vi "tui_Datalog Tag Subset Editor.vi"() -> ()   [LabVIEW 2012]
doc: "Edits subsets of the collection of tags in a logging database. Tag subsets allow related tags to be grouped. The subsets are ordered. It is possible to reorder the tags in a subset by dragging the items of the \"tags\" list that displays them. Several user interface windows that display information of multiple tags allow these tags to be quickly specified through selection of a subset.\n\nNote that subset definitions are automatically kept in sync with changes to the logging database: when tags that occur in subsets are deleted or renamed, the affected subsets will be updated accordingly. When this occurs while you are editing subsets, the editor will refuse to save any changes made relative to outdated subsets."
uses:
  served/DataLog Database Infos_srv.ctl
  served/DataLog Databases_srv.ctl
  typedefs/t_DataLog Tag Subset Editor States.ctl
  library/typedefs/t_Library Session Methods.ctl
  typedefs/t_DataLog Tag Info List Methods.ctl
  typedefs/t_Datalog Datebase Modes.ctl
  clientsrv/typedefs/t_ClientSrv Access Levels.ctl
panel:
  in  "reload subsets":bool
  in  "new subset":bool
  in  "rename subset":bool
  in  "delete subset":bool
  in  "sort subsets":bool
  in  "subsets":i32(listbox)
  in  "tags":i32(listbox)
  in  "add tag":bool
  in  "add multiple tags":bool
  in  "remove tag":bool
  in  "sort tags":bool
  out "databases":T1
  in  "database":i32(ring)
  in  "save subsets":bool
  in  "exit":bool
  out "database infos":T2
  in  "undo":bool
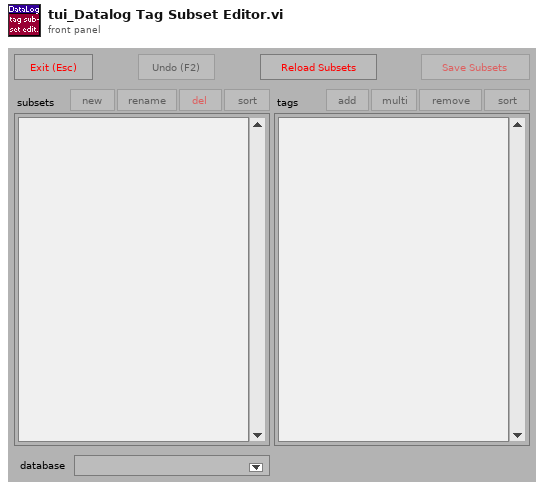
[diagram p1: front panel]
types:
  T1 = typedef "DataLog Databases_srv.ctl" = refnum<vi>
  T2 = typedef "DataLog Database Infos_srv.ctl" = refnum<vi>
  T3 = typedef "t_DataLog Tag Subset Editor States.ctl" = enum16{"empty queue", "set database", "load subsets", "save subsets", "new subset", "rename subset", "delete subset", "sort subsets", "add tag", "add tags", "remove tag", "sort tags", "update lists", "ablement", "resize", "initialize", "init refs", "init databases", "init access", "init persist", "cleanup", "stop"}
  T4 = typedef "t_Library Session Methods.ctl" = enum16{"run", "get arg", "set arg", "delist", "cleanup?", "start session", "stop session", "list empty?"}
  T5 = typedef "t_DataLog Tag Info List Methods.ctl" = enum16{"initialize", "create", "create empty", "rename", "delete", "test tag", "get", "get by name", "get default", "get list", "get path", "get subsets", "set subsets", "set config", "set capacity", "#tags", "go live", "set unlocked", "set mirrored"}
  T6 = typedef "t_Datalog Datebase Modes.ctl" = enum16{"locked", "unlocked", "live", "mirrored"}
  T7 = typedef "t_ClientSrv Access Levels.ctl" = enum16{"observer", "operator", "local"}
  T8 = typedef "t_DataLog Tag Subset.ctl" = cluster{"name":string, "tags":string[]}
  T9 = typedef "eventvkey.ctl" = enum16{"ASCII", "Enter", "Return", "Shift", "Ctrl", "Alt", "Cmd", "Opt", "Caps", "NumLock", "Clear", "Break", "Up", "Down", "Left", "Right", "Insert", "Delete", "Home", "End", "PageUp", "PageDown", "Escape", "Help", "Pause", "ScrollLock", "F1", "F2", "F3", "F4", "F5", "F6", "F7", "F8", "F9", "F10", "F11", "F12", "F13", "F14", "F15", "F16", "F17", "F18", "F19", "F20", "F21", "F22", "F23", "F24", "Play", "VolumeUp", "VolumeDown", "Mute", "Two Byte Char"}
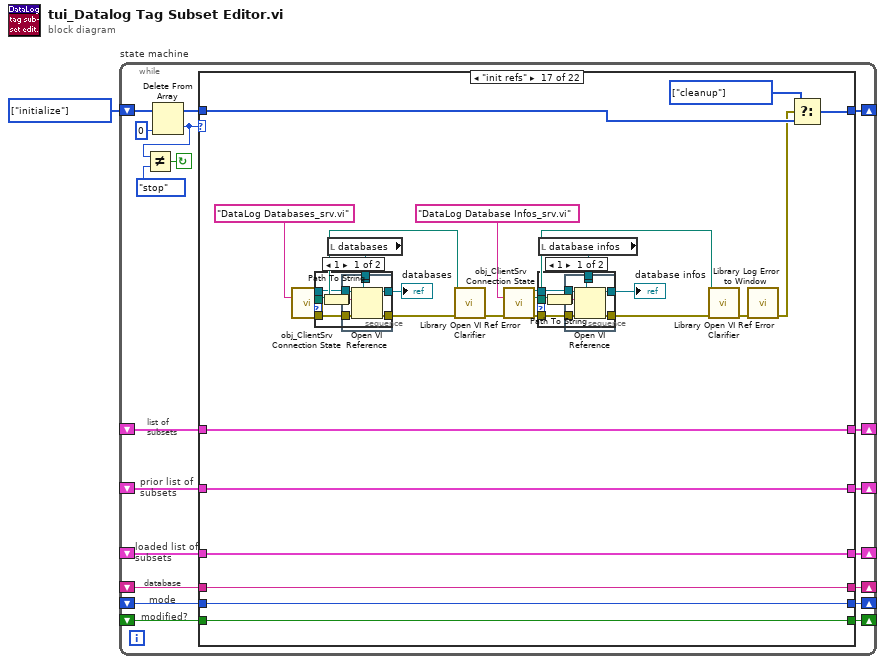
[diagram p0: block diagram]
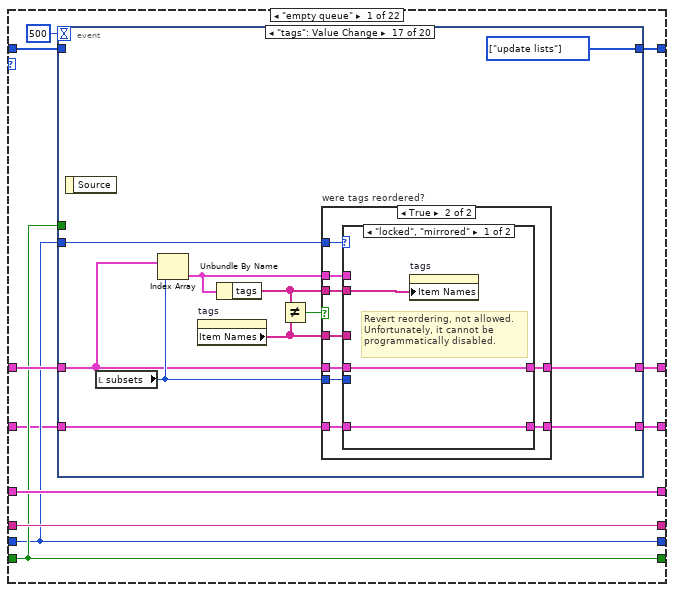
[diagram p2: hidden frame]
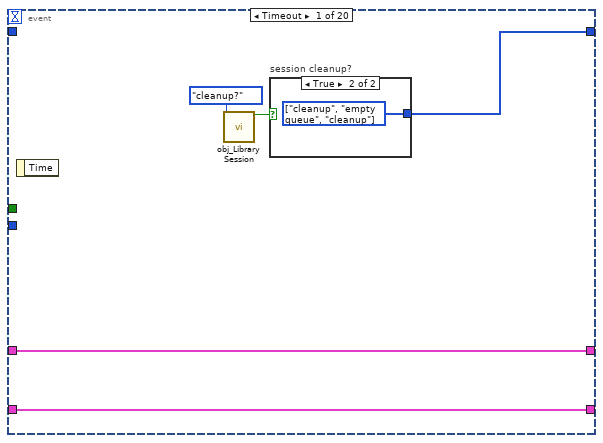
[diagram p3: hidden frame]
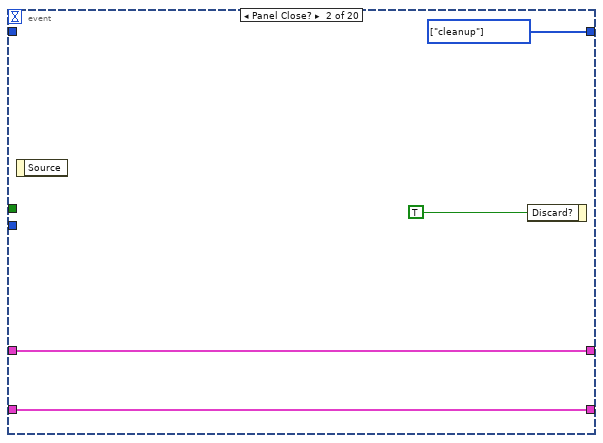
[diagram p5: hidden frame]
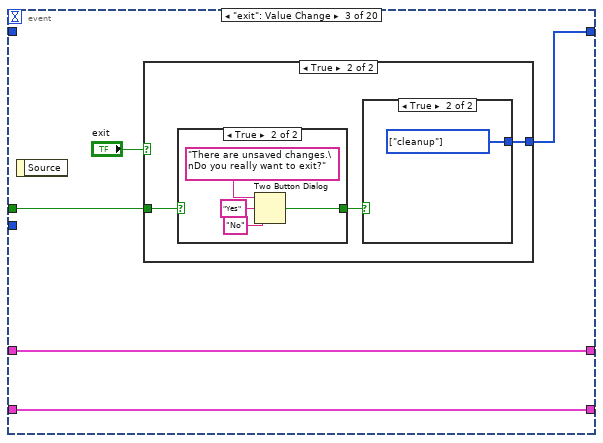
[diagram p6: hidden frame]
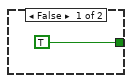
[diagram p8: hidden frame]
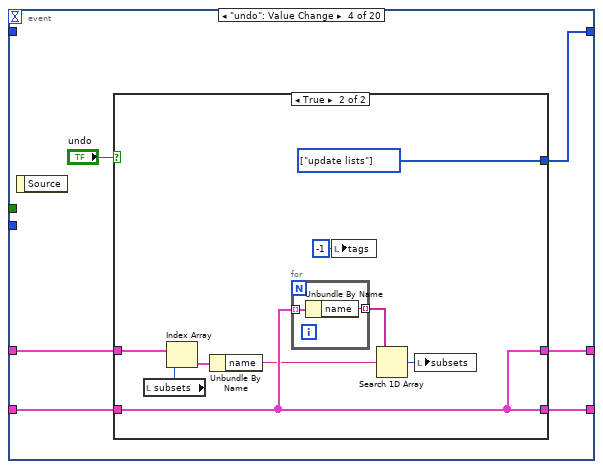
[diagram p10: hidden frame]
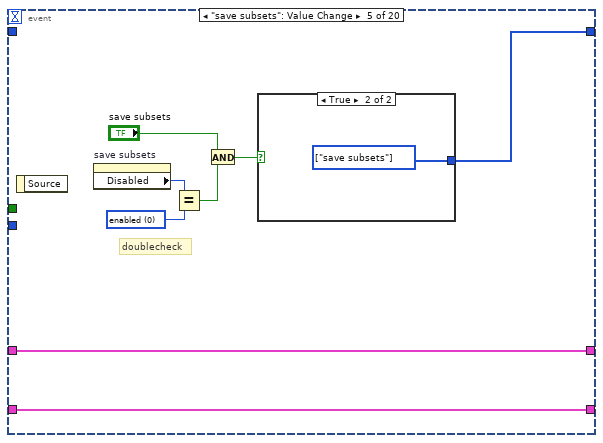
[diagram p12: hidden frame]
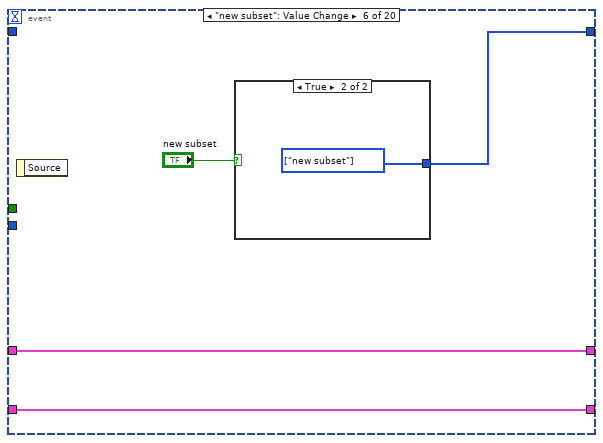
[diagram p14: hidden frame]
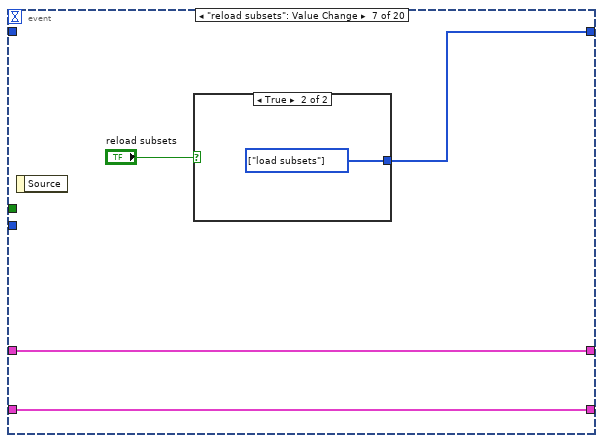
[diagram p16: hidden frame]
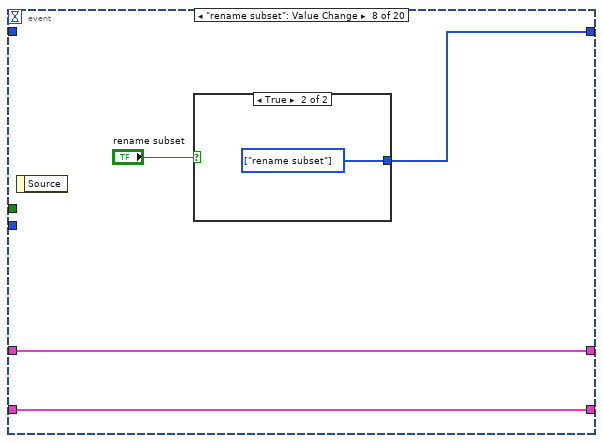
[diagram p18: hidden frame]
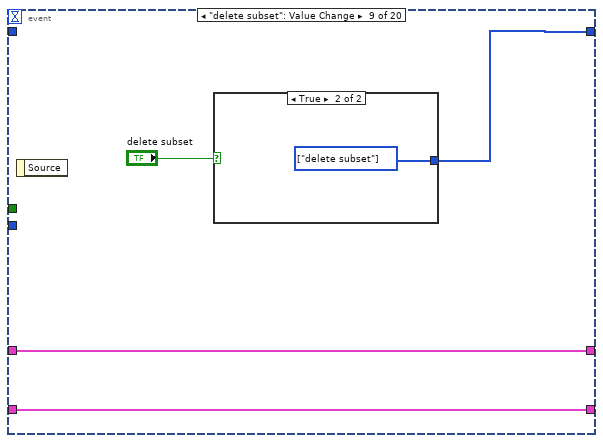
[diagram p20: hidden frame]
diagram:
  w1 = T3[] [enum."initialize"] items=["empty queue", "set database", "load subsets", "save subsets", "new subset", "rename subset", "delete subset", "sort subsets", "add tag", "add tags", "remove tag", "sort tags", "update lists", "ablement", "resize", "initialize", "init refs", "init databases", "init access", "init persist", "cleanup", "stop"] ("Array Constant")
  n1 = while "state machine" {
    shift-left: w1 -> [w17]
    shift-right: [w20] -> _
    shift-right: [w14] -> _
    shift-left: _ -> [w13]
    shift-right: [w10] -> _
    shift-left: _ -> [w11]
    shift-right: [w9] -> _
    shift-left: _ -> [w8]
    shift-right: [w7] -> _
    shift-left: _ -> [w6]
    shift-right: [w5] -> _
    shift-left: _ -> [w4]
    shift-right: [w3] -> _
    shift-left: _ -> [w2]
    stop <- w19 continue-if-true
    # "prior list of\nsubsets"
    # "modified?"
    # "mode"
    # "loaded list of\nsubsets"
    # "database"
    # "list of\nsubsets"
    n2 = Delete From Array(array=w17, index=0) -> (deleted portion=w12:T3, array with subset deleted=w16:T3[])  [unwired: 1 in]
    n3 = Not Equal?(x=w12, y=t_DataLog_Tag_Subset_Editor_States."stop" ("states")) -> (x != y?=w19:bool)
    n4 = case "Case" shown="\"init refs\"" w12 {
      tunnel: [w31 w227 w239 w286 w318 w374 w426 w437 w461 w504 w569 w589 w606 w657 w662 w733 w784 w837 w855 w859 w883 w890] -> w20
      tunnel: w16 -> [w29 w227 w240 w287 w319 w375 w427 w438 w462 w505 w570 w593 w613 w657 w662 _ w783 w827 w854 w865 _ w890]
      tunnel: [w27 w226 w236 w270 w320 w376 w428 w434 w469 w512 w556 w573 w603 w628 w661 w732 w781 w839 w857 w867 w881 w889] -> w14
      tunnel: w13 -> [w28 w226 _ w270 w325 w369 w429 w432 w470 w513 w558 w572 w603 w628 w661 w732 w781 w839 w857 w867 w881 w889]
      tunnel: w11 -> [w26 _ w235 w276 w317 w373 w425 w443 w460 w503 w568 w584 w608 w656 w666 w731 w777 w828 w849 w864 w876 w888]
      tunnel: [w26 w220 w235 w276 w317 w373 w425 w443 w460 w503 w568 w584 w608 w656 w666 w731 w777 w828 w849 w864 w876 w888] -> w10
      tunnel: [w25 w230 w236 w289 w316 w372 w424 w442 w466 w509 w566 w583 w604 w655 w665 w730 w774 w834 w852 w863 w873 w887] -> w9
      tunnel: w8 -> [w25 w230 _ w277 w316 w372 w424 w442 w466 w509 w566 w583 w604 w655 w665 w730 w774 w834 w852 w863 w873 w887]
      tunnel: [w23 w229 w241 w291 w315 w371 w423 w441 w465 w508 w565 w582 w607 w654 w664 w729 w773 w833 w851 w862 w872 w886] -> w7
      tunnel: w6 -> [w23 w229 _ w291 w315 w371 w423 w441 w465 w508 w565 w582 w607 w654 w664 w729 w773 w833 w851 w862 w872 w886]
      tunnel: [w24 w228 FALSE w290 w314 w370 w422 w440 w464 w507 w564 w581 w600 w646 w663 w728 w772 w832 w850 w861 w871 w885] -> w5
      tunnel: w4 -> [w24 w228 w237 w290 w314 w370 w422 w440 w464 w507 w564 w581 w602 w646 w663 w728 w772 w832 w850 w861 w871 w885]
      tunnel: [w21 w225 w236 w273 w313 w363 w420 w435 w459 w502 w560 w575 w599 w630 w660 w727 w771 w831 w846 w860 w868 w884] -> w3
      tunnel: w2 -> [w22 w225 _ w271 w312 w362 w421 w431 w458 w501 w559 w574 w599 w630 w660 w727 w771 w831 w846 w860 w868 w884]
      frame "empty queue" {
        n5 = event shown="[16] \"tags\": Value Change" {
          selector: _ -> [_ _ _ _ _ _ _ _ _ _ _ _ _ _ _ _ _ _ _ _]
          dyn-events: _ -> [_ _ _ _ _ _ _ _ _ _ _ _ _ _ _ _ _ _ _ _]
          timeout: 500 -> [_ _ _ _ _ _ _ _ _ _ _ _ _ _ _ _ _ _ _ _]
          tunnel: [w36 w41 w46 w61 w82 w87 w92 w97 w102 w107 w112 w117 w121 w126 w133 w150 w181 _ _ w217] -> w31
          tunnel: w29 -> [_ _ _ _ _ _ _ _ _ _ _ _ _ _ _ _ _ _ _ _]
          tunnel: w28 -> [w33 w39 w45 w56 w81 w86 w91 w96 w101 w106 w111 w116 w122 w127 w134 w147 w182 w207 w213 w219]
          tunnel: [w33 w39 w45 w59 w81 w86 w91 w96 w101 w106 w111 w116 w122 w127 w134 w145 w184 w207 w213 w219] -> w27
          tunnel: w24 -> [_ _ w43 _ _ _ _ _ _ _ _ _ _ _ w132 _ _ _ _ _]
          tunnel: w23 -> [_ _ _ _ _ _ _ _ _ _ _ _ _ _ _ w144 w176 _ _ _]
          tunnel: w22 -> [w32 w38 w42 w58 w80 w84 w89 w94 w99 w104 w109 w114 w119 w124 w129 w141 w174 w206 w212 w218]
          tunnel: [w32 w38 w42 w57 w80 w84 w89 w94 w99 w104 w109 w114 w119 w124 w129 w142 w175 w206 w212 w218] -> w21
          event Timeout {
            n6 = event-data() -> ()  [unwired: 1 in, 1 out]
            n7 = call "obj_Library Session.vi"("method"=t_Library_Session_Methods."cleanup?") -> ("cleanup/empty?"=w35:bool)  [unwired: 11 in, 3 out]
            n8 = case "session cleanup?" shown="True" w35 {
              tunnel: [_ w37] -> w36
              frame False {
              }
              frame True {
                w37 = T3[] [enum."cleanup", enum."empty queue", enum."cleanup"] items=["empty queue", "set database", "load subsets", "save subsets", "new subset", "rename subset", "delete subset", "sort subsets", "add tag", "add tags", "remove tag", "sort tags", "update lists", "ablement", "resize", "initialize", "init refs", "init databases", "init access", "init persist", "cleanup", "stop"] ("Array Constant")
              }
            }
          }
          event Panel Close? {
            w41 = T3[] [enum."cleanup"] items=["empty queue", "set database", "load subsets", "save subsets", "new subset", "rename subset", "delete subset", "sort subsets", "add tag", "add tags", "remove tag", "sort tags", "update lists", "ablement", "resize", "initialize", "init refs", "init databases", "init access", "init persist", "cleanup", "stop"] ("Array Constant")
            n9 = event-data() -> ()  [unwired: 1 in, 1 out]
            n10 = event-data("Discard?"=TRUE) -> ()  [unwired: 1 in, 1 out]
          }
          event "exit": Value Change {
            n11 = event-data() -> ()  [unwired: 1 in, 1 out]
            n12 = case shown="True" "exit" {
              tunnel: [_ w49] -> w46
              tunnel: w43 -> [_ w48]
              frame False {
              }
              frame True {
                n13 = case shown="True" w48 {
                  tunnel: [TRUE w53] -> w47
                  frame False {
                  }
                  frame True {
                    n14 = Two Button Dialog(message="There are unsaved changes.\nDo you really want to exit?", 1:"No" ("F button name (\"Cancel\")"), 2:"Yes" ("T button name (\"OK\")")) -> (T button?=w53:bool)
                  }
                }
                n15 = case shown="True" w47 {
                  tunnel: [_ w55] -> w49
                  frame False {
                  }
                  frame True {
                    w55 = T3[] [enum."cleanup"] items=["empty queue", "set database", "load subsets", "save subsets", "new subset", "rename subset", "delete subset", "sort subsets", "add tag", "add tags", "remove tag", "sort tags", "update lists", "ablement", "resize", "initialize", "init refs", "init databases", "init access", "init persist", "cleanup", "stop"] ("Array Constant")
                  }
                }
              }
            }
          }
          event "undo": Value Change {
            n16 = event-data() -> ()  [unwired: 1 in, 1 out]
            n17 = case shown="True" "undo" {
              tunnel: [_ w72] -> w61
              tunnel: [w63 w68] -> w59
              tunnel: w58 -> [w62 w68]
              tunnel: [w62 w68] -> w57
              tunnel: w56 -> [w63 w71]
              frame False {
              }
              frame True {
                w72 = T3[] [enum."update lists"] items=["empty queue", "set database", "load subsets", "save subsets", "new subset", "rename subset", "delete subset", "sort subsets", "add tag", "add tags", "remove tag", "sort tags", "update lists", "ablement", "resize", "initialize", "init refs", "init databases", "init access", "init persist", "cleanup", "stop"] ("Array Constant")
                n18 = local read "subsets"() -> (w70:i32)
                n19 = Index Array(array=w71, index=w70) -> (element=w69:T8)
                n20 = Unbundle By Name(w69) -> ("name"=w66:string)
                n21 = for {
                  tunnel: w68 -> [w74] mode=indexing
                  tunnel: [w73] -> w67 mode=indexing
                  n22 = Unbundle By Name(w74) -> ("name"=w73:string)
                }
                n23 = local write "tags"(-1 ("tags")) -> ()
                n24 = Search 1D Array(1D array=w67, element=w66) -> (index of element=w65:i32)  [unwired: 1 in]
                n25 = local write "subsets"(w65) -> ()
              }
            }
          }
          event "save subsets": Value Change {
            w79 = u8 0 items=["enabled", "disabled", "grayed"] ("disabled state")
            # "doublecheck"
            n26 = event-data() -> ()  [unwired: 1 in, 1 out]
            n27 = property on="save subsets" class="Bool"() -> ("Disabled"=w78:u8)  [unwired: 2 in, 2 out]
            n28 = Equal?(x=w78, y=w79) -> (x = y?=w76:bool)
            n29 = And(x="save subsets", y=w76) -> (x .and. y?=w75:bool)
            n30 = case shown="True" w75 {
              tunnel: [_ w83] -> w82
              frame False {
              }
              frame True {
                w83 = T3[] [enum."save subsets"] items=["empty queue", "set database", "load subsets", "save subsets", "new subset", "rename subset", "delete subset", "sort subsets", "add tag", "add tags", "remove tag", "sort tags", "update lists", "ablement", "resize", "initialize", "init refs", "init databases", "init access", "init persist", "cleanup", "stop"] ("Array Constant")
              }
            }
          }
          event "new subset": Value Change {
            n31 = event-data() -> ()  [unwired: 1 in, 1 out]
            n32 = case shown="True" "new subset" {
              tunnel: [_ w88] -> w87
              frame False {
              }
              frame True {
                w88 = T3[] [enum."new subset"] items=["empty queue", "set database", "load subsets", "save subsets", "new subset", "rename subset", "delete subset", "sort subsets", "add tag", "add tags", "remove tag", "sort tags", "update lists", "ablement", "resize", "initialize", "init refs", "init databases", "init access", "init persist", "cleanup", "stop"] ("Array Constant")
              }
            }
          }
          event "reload subsets": Value Change {
            n33 = event-data() -> ()  [unwired: 1 in, 1 out]
            n34 = case shown="True" "reload subsets" {
              tunnel: [_ w93] -> w92
              frame False {
              }
              frame True {
                w93 = T3[] [enum."load subsets"] items=["empty queue", "set database", "load subsets", "save subsets", "new subset", "rename subset", "delete subset", "sort subsets", "add tag", "add tags", "remove tag", "sort tags", "update lists", "ablement", "resize", "initialize", "init refs", "init databases", "init access", "init persist", "cleanup", "stop"] ("Array Constant")
              }
            }
          }
          event "rename subset": Value Change {
            n35 = event-data() -> ()  [unwired: 1 in, 1 out]
            n36 = case shown="True" "rename subset" {
              tunnel: [_ w98] -> w97
              frame False {
              }
              frame True {
                w98 = T3[] [enum."rename subset"] items=["empty queue", "set database", "load subsets", "save subsets", "new subset", "rename subset", "delete subset", "sort subsets", "add tag", "add tags", "remove tag", "sort tags", "update lists", "ablement", "resize", "initialize", "init refs", "init databases", "init access", "init persist", "cleanup", "stop"] ("Array Constant")
              }
            }
          }
          event "delete subset": Value Change {
            n37 = event-data() -> ()  [unwired: 1 in, 1 out]
            n38 = case shown="True" "delete subset" {
              tunnel: [_ w103] -> w102
              frame False {
              }
              frame True {
                w103 = T3[] [enum."delete subset"] items=["empty queue", "set database", "load subsets", "save subsets", "new subset", "rename subset", "delete subset", "sort subsets", "add tag", "add tags", "remove tag", "sort tags", "update lists", "ablement", "resize", "initialize", "init refs", "init databases", "init access", "init persist", "cleanup", "stop"] ("Array Constant")
              }
            }
          }
          event "remove tag": Value Change {
            n39 = event-data() -> ()  [unwired: 1 in, 1 out]
            n40 = case shown="True" "remove tag" {
              tunnel: [_ w108] -> w107
              frame False {
              }
              frame True {
                w108 = T3[] [enum."remove tag"] items=["empty queue", "set database", "load subsets", "save subsets", "new subset", "rename subset", "delete subset", "sort subsets", "add tag", "add tags", "remove tag", "sort tags", "update lists", "ablement", "resize", "initialize", "init refs", "init databases", "init access", "init persist", "cleanup", "stop"] ("Array Constant")
              }
            }
          }
          event "add tag": Value Change {
            n41 = event-data() -> ()  [unwired: 1 in, 1 out]
            n42 = case shown="True" "add tag" {
              tunnel: [_ w113] -> w112
              frame False {
              }
              frame True {
                w113 = T3[] [enum."add tag"] items=["empty queue", "set database", "load subsets", "save subsets", "new subset", "rename subset", "delete subset", "sort subsets", "add tag", "add tags", "remove tag", "sort tags", "update lists", "ablement", "resize", "initialize", "init refs", "init databases", "init access", "init persist", "cleanup", "stop"] ("Array Constant")
              }
            }
          }
          event "add multiple tags": Value Change {
            n43 = event-data() -> ()  [unwired: 1 in, 1 out]
            n44 = case shown="True" "add multiple tags" {
              tunnel: [_ w118] -> w117
              frame False {
              }
              frame True {
                w118 = T3[] [enum."add tags"] items=["empty queue", "set database", "load subsets", "save subsets", "new subset", "rename subset", "delete subset", "sort subsets", "add tag", "add tags", "remove tag", "sort tags", "update lists", "ablement", "resize", "initialize", "init refs", "init databases", "init access", "init persist", "cleanup", "stop"] ("Array Constant")
              }
            }
          }
          event "sort tags": Value Change {
            n45 = event-data() -> ()  [unwired: 1 in, 1 out]
            n46 = case shown="True" "sort tags" {
              tunnel: [_ w123] -> w121
              frame False {
              }
              frame True {
                w123 = T3[] [enum."sort tags"] items=["empty queue", "set database", "load subsets", "save subsets", "new subset", "rename subset", "delete subset", "sort subsets", "add tag", "add tags", "remove tag", "sort tags", "update lists", "ablement", "resize", "initialize", "init refs", "init databases", "init access", "init persist", "cleanup", "stop"] ("Array Constant")
              }
            }
          }
          event "sort subsets": Value Change {
            n47 = event-data() -> ()  [unwired: 1 in, 1 out]
            n48 = case shown="True" "sort subsets" {
              tunnel: [_ w128] -> w126
              frame False {
              }
              frame True {
                w128 = T3[] [enum."sort subsets"] items=["empty queue", "set database", "load subsets", "save subsets", "new subset", "rename subset", "delete subset", "sort subsets", "add tag", "add tags", "remove tag", "sort tags", "update lists", "ablement", "resize", "initialize", "init refs", "init databases", "init access", "init persist", "cleanup", "stop"] ("Array Constant")
              }
            }
          }
          event "database": Value Change {
            n49 = event-data() -> ("OldVal"=w130:i32)  [unwired: 1 in]
            n50 = case shown="False" w132 {
              tunnel: [TRUE w138] -> w131
              frame False {
              }
              frame True {
                n51 = Two Button Dialog(message="You have selected a new database\nbut the prior database has unsaved\nsubset changes. If you proceed,\nthese changes will be discarded.", 2:"Proceed" ("T button name (\"OK\")")) -> (T button?=w138:bool)  [unwired: 1 in]
              }
            }
            n52 = case shown="True" w131 {
              tunnel: [_ w140] -> w133
              tunnel: w130 -> [w139 _]
              frame False {
                n53 = local write "database"(w139) -> ()
              }
              frame True {
                w140 = T3[] [enum."set database", enum."load subsets"] items=["empty queue", "set database", "load subsets", "save subsets", "new subset", "rename subset", "delete subset", "sort subsets", "add tag", "add tags", "remove tag", "sort tags", "update lists", "ablement", "resize", "initialize", "init refs", "init databases", "init access", "init persist", "cleanup", "stop"] ("Array Constant")
              }
            }
          }
          event "subsets": Value Change {
            w150 = T3[] [enum."update lists"] items=["empty queue", "set database", "load subsets", "save subsets", "new subset", "rename subset", "delete subset", "sort subsets", "add tag", "add tags", "remove tag", "sort tags", "update lists", "ablement", "resize", "initialize", "init refs", "init databases", "init access", "init persist", "cleanup", "stop"] ("Array Constant")
            n54 = event-data() -> ()  [unwired: 1 in, 1 out]
            n55 = for {
              tunnel: w147 -> [w173] mode=indexing
              tunnel: [w172] -> w146 mode=indexing
              n56 = Unbundle By Name(w173) -> ("name"=w172:string)
            }
            n57 = property on="subsets" class="LstBox (strict)"() -> ("Item Names"=w148:string[])  [unwired: 2 in, 2 out]
            n58 = Not Equal?(x=w148, y=w146) -> (x != y?=w149:bool)
            n59 = case "were subsets reordered?" shown="True" w149 {
              tunnel: w148 -> [_ w159]
              tunnel: w147 -> [w152 w157]
              tunnel: w146 -> [_ w158]
              tunnel: [w152 w156] -> w145
              tunnel: w144 -> [_ w155]
              tunnel: [w151 w154] -> w142
              tunnel: w141 -> [w151 w153]
              frame False {
              }
              frame True {
                n60 = case shown="\"locked\", \"mirrored\"" w155 {
                  tunnel: w159 -> [_ w166]
                  tunnel: w158 -> [w161 w165]
                  tunnel: w157 -> [w162 w163]
                  tunnel: [w162 w164] -> w156
                  tunnel: [w160 w163] -> w154
                  tunnel: w153 -> [w160 _]
                  frame "locked", "mirrored" {
                    # "Revert reordering, not allowed.\nUnfortunately, it cannot be\nprogrammatically disabled."
                    n61 = property on="subsets" class="LstBox (strict)"("Item Names"=w161) -> ()  [unwired: 2 in, 2 out]
                  }
                  frame "unlocked", "live" {
                    n62 = for {
                      tunnel: w166 -> [w170] mode=indexing
                      tunnel: w165 -> [w171]
                      tunnel: w163 -> [w168]
                      tunnel: [w167] -> w164 mode=indexing
                      n63 = Search 1D Array(1D array=w171, element=w170) -> (index of element=w169:i32)  [unwired: 1 in]
                      n64 = Index Array(array=w168, index=w169) -> (element=w167:T8)
                    }
                  }
                }
              }
            }
            n65 = local write "tags"(-1 ("list of tag subsets")) -> ()
          }
          event "tags": Value Change {
            w181 = T3[] [enum."update lists"] items=["empty queue", "set database", "load subsets", "save subsets", "new subset", "rename subset", "delete subset", "sort subsets", "add tag", "add tags", "remove tag", "sort tags", "update lists", "ablement", "resize", "initialize", "init refs", "init databases", "init access", "init persist", "cleanup", "stop"] ("Array Constant")
            n66 = event-data() -> ()  [unwired: 1 in, 1 out]
            n67 = local read "subsets"() -> (w183:i32)
            n68 = Index Array(array=w182, index=w183) -> (element=w179:T8)
            n69 = property on="tags" class="LstBox (strict)"() -> ("Item Names"=w178:string[])  [unwired: 2 in, 2 out]
            n70 = Unbundle By Name(w179) -> ("tags"=w177:string[])
            n71 = Not Equal?(x=w177, y=w178) -> (x != y?=w180:bool)
            n72 = case "were tags reordered?" shown="True" w180 {
              tunnel: [w186 w195] -> w184
              tunnel: w183 -> [_ w194]
              tunnel: w182 -> [w186 w193]
              tunnel: w179 -> [_ w192]
              tunnel: w178 -> [_ w191]
              tunnel: w177 -> [_ w190]
              tunnel: w176 -> [_ w189]
              tunnel: [w185 w188] -> w175
              tunnel: w174 -> [w185 w187]
              frame False {
              }
              frame True {
                n73 = case shown="\"locked\", \"mirrored\"" w189 {
                  tunnel: [w198 w204] -> w195
                  tunnel: w194 -> [_ w203]
                  tunnel: w193 -> [w198 w199]
                  tunnel: w192 -> [_ w201]
                  tunnel: w191 -> [_ w200]
                  tunnel: w190 -> [w197 _]
                  tunnel: [w196 w199] -> w188
                  tunnel: w187 -> [w196 _]
                  frame "locked", "mirrored" {
                    # "Revert reordering, not allowed.\nUnfortunately, it cannot be\nprogrammatically disabled."
                    n74 = property on="tags" class="LstBox (strict)"("Item Names"=w197) -> ()  [unwired: 2 in, 2 out]
                  }
                  frame "unlocked", "live" {
                    n75 = Bundle By Name(cluster=w201, "tags"=w200) -> (w202:T8)
                    n76 = Replace Array Subset(array=w199, new element=w202, index=w203) -> (w204:T8[])
                  }
                }
              }
            }
          }
          event Key Down? {
            n77 = event-data() -> ("VKey"=w205:T9)  [unwired: 1 in]
            n78 = call <vilib>:"compatReturnToEnter.vi"("VKey"=w205) -> ("VKey"=w209:T9)
            n79 = case shown="\"F1\"" w209 {
              tunnel: [_ TRUE ("Discard?")] -> w208
              frame Default {
              }
              frame "F1" {
                n80 = call "Library Show Help.vi"() -> ()  [unwired: 1 in]
              }
            }
            n81 = event-data("Discard?"=w208) -> ()  [unwired: 1 in, 1 out]
          }
          event event type 5.0.x8000000b {
            n82 = event-data() -> ("VKey"=w211:T9)  [unwired: 1 in]
            n83 = call <vilib>:"compatReturnToEnter.vi"("VKey"=w211) -> ("VKey"=w215:T9)
            n84 = case shown="\"F1\"" w215 {
              tunnel: [_ TRUE ("Discard?")] -> w214
              frame Default {
              }
              frame "F1" {
              }
            }
            n85 = event-data("Discard?"=w214) -> ()  [unwired: 1 in, 1 out]
          }
          event Panel Resize {
            w217 = T3[] [enum."resize"] items=["empty queue", "set database", "load subsets", "save subsets", "new subset", "rename subset", "delete subset", "sort subsets", "add tag", "add tags", "remove tag", "sort tags", "update lists", "ablement", "resize", "initialize", "init refs", "init databases", "init access", "init persist", "cleanup", "stop"] ("Array Constant")
            n86 = event-data() -> ()  [unwired: 1 in, 1 out]
          }
        }
      }
      frame "set database" {
        n87 = property on="database" class="Ring (strict)"() -> ("Strings []"=w221:string[])  [unwired: 2 in, 2 out]
        n88 = Index Array(array=w221, index="database") -> (element=w222:string)
        n89 = Empty String/Path?(string/path=w222) -> (empty?=w223:bool)
        n90 = case shown="True" w223 {
          tunnel: w221 -> [_ w234]
          tunnel: w222 -> [w231 _]
          tunnel: [w231 w233] -> w220
          frame False {
          }
          frame True {
            w232 = 0 ("index")
            n91 = Index Array(array=w234, index=w232) -> (element=w233:string)
            n92 = local write "database"(w232) -> ()
          }
        }
      }
      frame "load subsets" {
        n93 = call "obj_ClientSrv Client Access State.vi"() -> ("certificate"=w246:string, "error out"=w250:errorcluster)  [unwired: 14 in]
        n94 = local read "database infos"() -> (w247:T2)
        n95 = call-by-ref "?"(reference=w247, error in=w250, "method"=t_DataLog_Tag_Info_List_Methods."get subsets", "certificate in"=w246, "database (current)"=w235) -> (error out=w249:errorcluster, "mode"=w244:T6, "subsets out"=w242:T8[], 15:"error out"=w248:errorcluster)  [unwired: 7 in, 4 out]
        n96 = call "Library Remote Call Error Merger.vi"("call by reference node error"=w249, "called VI error (no error)"=w248) -> ("error out"=w243:errorcluster)  [unwired: 13 in]
        n97 = case shown="No Error" w243 {
          selector: w243 -> [_ w268]
          tunnel: w244 -> [w259 _]
          tunnel: w242 -> [w258 _]
          tunnel: [w258 _] -> w236
          tunnel: [w257 t_Datalog_Datebase_Modes."locked" ("mode")] -> w241
          tunnel: w240 -> [w256 _]
          tunnel: [w255 w267] -> w239
          tunnel: w237 -> [w251 _]
          frame No Error {
            n98 = case shown="\"locked\", \"mirrored\"" w259 {
              selector: w259 -> [w262 w266]
              tunnel: [w262 w266] -> w257
              tunnel: [-1 ("list of tag subsets") 0 ("list of tag subsets")] -> w252
              frame "locked", "mirrored" {
                n99 = Format Into String(format string="Database is %s. Can view\nbut not edit its tag subsets.", w262) -> (resulting string=w263:string)  [unwired: 2 in, 1 out]
                n100 = One Button Dialog(message=w263) -> ()  [unwired: 1 in, 1 out]
              }
              frame "unlocked", "live" {
              }
            }
            n101 = case shown="True" w251 {
              frame False {
              }
              frame True {
                n102 = property class="VI"("Front Panel Window:Title"="Tag Subset Editor") -> ()  [unwired: 2 in, 2 out]
              }
            }
            n103 = local write "tags"(-1 ("list of tag subsets")) -> ()
            n104 = local write "subsets"(w252) -> ()
            n105 = Build Array (concatenate)(t_DataLog_Tag_Subset_Editor_States."update lists" ("states"), w256) -> (w255:T3[])
          }
          frame Error {
            w267 = T3[] [enum."cleanup"] items=["empty queue", "set database", "load subsets", "save subsets", "new subset", "rename subset", "delete subset", "sort subsets", "add tag", "add tags", "remove tag", "sort tags", "update lists", "ablement", "resize", "initialize", "init refs", "init databases", "init access", "init persist", "cleanup", "stop"] ("Array Constant")
            n106 = call "Library Log Error to Window.vi"("error in (no error)"=w268) -> ()  [unwired: 13 in, 2 out]
          }
        }
      }
      frame "save subsets" {
        n107 = local read "database infos"() -> (w282:T2)
        n108 = call "obj_ClientSrv Client Access State.vi"() -> ("certificate"=w284:string, "error out"=w283:errorcluster)  [unwired: 14 in]
        n109 = call-by-ref "?"(reference=w282, error in=w283, "method"=t_DataLog_Tag_Info_List_Methods."get subsets", "certificate in"=w284, "database (current)"=w276) -> (reference out=w281:T2, error out=w280:errorcluster, "subsets out"=w278:T8[], 15:"error out"=w279:errorcluster)  [unwired: 7 in, 4 out]
        n110 = Equal?(x=w278, y=w277) -> (x = y?=w274:bool)
        n111 = call "Library Remote Call Error Merger.vi"("call by reference node error"=w280, "called VI error (no error)"=w279) -> ("error out"=w275:errorcluster)  [unwired: 13 in]
        n112 = case shown="No Error" w275 {
          selector: w275 -> [_ w311]
          tunnel: w270 -> [w296 _]
          tunnel: [w295 w310] -> w272
          tunnel: w281 -> [w294 _]
          tunnel: w276 -> [w293 _]
          tunnel: w274 -> [w292 _]
          frame No Error {
            n113 = case "subsets remained unchanged while editing?" shown="True" w292 {
              tunnel: w293 -> [_ w309]
              tunnel: w296 -> [_ w301]
              tunnel: [TRUE w300] -> w295
              tunnel: w294 -> [_ w299]
              frame False {
                n114 = One Button Dialog(message="Cannot save changes. While editing, the\nsubsets of the database were modified.\nThis can happen when tags are renamed\nor deleted while editing, or another user\nhas edited subsets in the mean time.\n\nFirst reload the subsets to make changes\nagainst to the current definitions.") -> ()  [unwired: 1 in, 1 out]
              }
              frame True {
                n115 = call "obj_ClientSrv Client Access State.vi"("access level (observer)"=t_ClientSrv_Access_Levels."operator") -> ("certificate"=w303:string, "error out"=w308:errorcluster)  [unwired: 13 in]
                n116 = call-by-ref "?"(reference=w299, error in=w308, "method"=t_DataLog_Tag_Info_List_Methods."set subsets", "subsets in"=w301, "certificate in"=w303, "database (current)"=w309) -> (error out=w307:errorcluster, 15:"error out"=w304:errorcluster)  [unwired: 6 in, 6 out]
                n117 = call "Library Remote Call Error Merger.vi"("call by reference node error"=w307, "called VI error (no error)"=w304) -> ("error out"=w306:errorcluster)  [unwired: 13 in]
                n118 = call "Library Log Error to Window.vi"("error in (no error)"=w306) -> ("error?"=w300:bool)  [unwired: 13 in, 1 out]
              }
            }
          }
          frame Error {
            n119 = call "Library Log Error to Window.vi"("error in (no error)"=w311) -> ("error?"=w310:bool)  [unwired: 13 in, 1 out]
          }
        }
        n120 = Build Array (concatenate)(t_DataLog_Tag_Subset_Editor_States."update lists" ("states"), w287) -> (w286:T3[])
        n121 = Select(t=w271, s=w272, f=w270) -> (s? t:f=w273:T8[])
        n122 = Select(t=w277, s=w272, f=w270) -> (s? t:f=w289:T8[])
      }
      frame "new subset" {
        n123 = call "ui_Library Query String.vi"("prompt"="Name the new tag subset") -> ("OKed?"=w324:bool, "string out"=w321:string)  [unwired: 13 in]
        n124 = Empty String/Path?(string/path=w321) -> (empty?=w323:bool)
        n125 = Compound Arithmetic op=AND(w324, invert w323) -> (w322:bool)
        n126 = case shown="True" w322 {
          tunnel: w325 -> [w328 w335]
          tunnel: w321 -> [_ w333]
          tunnel: [w328 w338] -> w320
          tunnel: w319 -> [w329 w337]
          tunnel: [w329 w336] -> w318
          tunnel: [w327 w331] -> w313
          tunnel: w312 -> [w327 w330]
          frame False {
          }
          frame True {
            n127 = for {
              tunnel: w335 -> [w344] mode=indexing
              shift-right: [w339] -> w332
              shift-left: FALSE -> [w343]
              tunnel: w333 -> [w341]
              n128 = Unbundle By Name(w344) -> ("name"=w342:string)
              n129 = Equal?(x=w341, y=w342) -> (x = y?=w340:bool)
              n130 = Or(x=w343, y=w340) -> (x .or. y?=w339:bool)
            }
            n131 = case "exists already?" shown="False" w332 {
              tunnel: w335 -> [w345 w361]
              tunnel: [w355 w361] -> w338
              tunnel: w333 -> [w352 w359]
              tunnel: w337 -> [w347 w360]
              tunnel: [w346 w360] -> w336
              tunnel: [w345 w356] -> w331
              tunnel: w330 -> [_ w356]
              frame False {
                n132 = Index Array(array=w345, index=0) -> (element=w353:T8)
                n133 = Bundle By Name(cluster=w353, "name"=w352, "tags"=string[] []) -> (w350:T8)
                n134 = Array Size(array=w345) -> (size(s)=w349:i32)
                n135 = Build Array (concatenate)(w345, w350) -> (w355:T8[])
                n136 = Build Array (concatenate)(t_DataLog_Tag_Subset_Editor_States."update lists" ("states"), w347) -> (w346:T3[])
                n137 = local write "subsets"(w349) -> ()
              }
              frame True {
                n138 = Format Into String(format string="Subset \"%s\" already exists.", w359) -> (resulting string=w357:string)  [unwired: 2 in, 1 out]
                n139 = One Button Dialog(message=w357) -> ()  [unwired: 1 in, 1 out]
              }
            }
          }
        }
      }
      frame "rename subset" {
        n140 = local read "subsets"() -> (w368:i32)
        n141 = Index Array(array=w369, index=w368) -> (element=w367:T8)
        n142 = Unbundle By Name(w367) -> ("name"=w365:string)
        n143 = call "ui_Library Query String.vi"("prompt"="Specify a new subset name", "string in (\"\")"=w365) -> ("OKed?"=w379:bool, "string out"=w366:string)  [unwired: 12 in]
        n144 = Equal?(x=w366, y=w365) -> (x = y?=w364:bool)
        n145 = Empty String/Path?(string/path=w366) -> (empty?=w378:bool)
        n146 = Compound Arithmetic op=AND(w379, invert w378, invert w364) -> (w377:bool)
        n147 = case "new name OKed?" shown="True" w377 {
          tunnel: w369 -> [w382 w390]
          tunnel: w366 -> [_ w388]
          tunnel: [w382 w393] -> w376
          tunnel: w375 -> [w383 w392]
          tunnel: [w383 w391] -> w374
          tunnel: w368 -> [_ w386]
          tunnel: [w381 w385] -> w363
          tunnel: w362 -> [w381 w384]
          frame False {
          }
          frame True {
            n148 = for {
              tunnel: w390 -> [w399] mode=indexing
              shift-right: [w394] -> w387
              shift-left: FALSE -> [w398]
              tunnel: w388 -> [w396]
              n149 = Unbundle By Name(w399) -> ("name"=w397:string)
              n150 = Equal?(x=w396, y=w397) -> (x = y?=w395:bool)
              n151 = Or(x=w398, y=w395) -> (x .or. y?=w394:bool)
            }
            n152 = case "exists already?" shown="False" w387 {
              tunnel: w390 -> [w400 w414]
              tunnel: [w403 w414] -> w393
              tunnel: w388 -> [w407 w412]
              tunnel: w392 -> [w405 w413]
              tunnel: [w404 w413] -> w391
              tunnel: w386 -> [w401 _]
              tunnel: [w400 w409] -> w385
              tunnel: w384 -> [_ w409]
              frame False {
                n153 = Index Array(array=w400, index=w401) -> (element=w408:T8)
                n154 = Bundle By Name(cluster=w408, "name"=w407) -> (w402:T8)
                n155 = Build Array (concatenate)(t_DataLog_Tag_Subset_Editor_States."update lists" ("states"), w405) -> (w404:T3[])
                n156 = Replace Array Subset(array=w400, new element=w402, index=w401) -> (w403:T8[])
              }
              frame True {
                n157 = Format Into String(format string="Subset \"%s\" already exists.", w412) -> (resulting string=w410:string)  [unwired: 2 in, 1 out]
                n158 = One Button Dialog(message=w410) -> ()  [unwired: 1 in, 1 out]
              }
            }
          }
        }
      }
      frame "delete subset" {
        n159 = local read "subsets"() -> (w430:i32)
        n160 = Delete From Array(array=w429, index=w430) -> (array with subset deleted=w428:T8[])  [unwired: 1 in, 1 out]
        n161 = Not Equal?(x=w428, y=w429) -> (x != y?=w418:bool)
        n162 = Array Size(array=w428) -> (size(s)=w415:i32)
        n163 = Select(t=w429, s=w418, f=w421) -> (s? t:f=w420:T8[])
        n164 = Decrement(x=w415) -> (x-1=w417:i32)
        n165 = Max & Min(x=w430, y=w417) -> (min(x,y)=w416:i32)  [unwired: 1 out]
        n166 = local write "subsets"(w416) -> ()
        n167 = Build Array (concatenate)(t_DataLog_Tag_Subset_Editor_States."update lists" ("states"), w427) -> (w426:T3[])
      }
      frame "sort subsets" {
        # "avoid LV7 bug"
        # "sort case independently"
        n168 = for {
          tunnel: w432 -> [w455] mode=indexing
          tunnel: [w454] -> w446 mode=indexing
          n169 = Unbundle By Name(w455) -> ("name"=w457:string)
          n170 = To Lower Case(string=w457) -> (all lower case string=w456:string)
          n171 = Bundle(w456, w455) -> (w454:cluster{string, T8})  [unwired: 1 in]
        }
        n172 = local read "subsets"() -> (w436:i32)
        n173 = Index Array(array=w432, index=w436) -> (element=w450:T8)
        n174 = Unbundle By Name(w450) -> ("name"=w448:string)
        n175 = Sort 1D Array(array=w446) -> (sorted array=w445:cluster{string, T8}[])
        n176 = Sort 1D Array(array=w445) -> (sorted array=w444:cluster{string, T8}[])
        n177 = for {
          tunnel: w444 -> [w453] mode=indexing
          tunnel: [w452] -> w434 mode=indexing
          tunnel: [w451] -> w449 mode=indexing
          n178 = Unbundle(w453) -> (w452:T8)  [unwired: 1 out]
          n179 = Unbundle By Name(w452) -> ("name"=w451:string)
        }
        n180 = Search 1D Array(1D array=w449, element=w448) -> (index of element=w447:i32)  [unwired: 1 in]
        n181 = Not Equal?(x=w434, y=w432) -> (x != y?=w433:bool)
        n182 = local write "subsets"(w447) -> ()
        n183 = Build Array (concatenate)(t_DataLog_Tag_Subset_Editor_States."update lists" ("states"), w438) -> (w437:T3[])
        n184 = Select(t=w432, s=w433, f=w431) -> (s? t:f=w435:T8[])
      }
      frame "add tag" {
        n185 = call "ui_DataLog Query Tag.vi"("prompt"="Select a tag to add", "database"=w460) -> ("OK?"=w468:bool, "tag"=w467:string)  [unwired: 12 in]
        n186 = case "OKed?" shown="True" w468 {
          tunnel: w470 -> [w473 w480]
          tunnel: [w473 w479] -> w469
          tunnel: w467 -> [_ w482]
          tunnel: w462 -> [w472 w477]
          tunnel: [w472 w476] -> w461
          tunnel: [w471 w475] -> w459
          tunnel: w458 -> [w471 w474]
          frame False {
          }
          frame True {
            n187 = local read "subsets"() -> (w478:i32)
            n188 = Index Array(array=w480, index=w478) -> (element=w481:T8)
            n189 = Unbundle By Name(w481) -> ("tags"=w484:string[])
            n190 = Search 1D Array(1D array=w484, element=w482) -> (index of element=w483:i32)  [unwired: 1 in]
            n191 = case shown="Default" w483 {
              tunnel: w484 -> [_ w493]
              tunnel: w482 -> [_ w500]
              tunnel: w481 -> [_ w499]
              tunnel: w480 -> [w487 w489]
              tunnel: [w487 w497] -> w479
              tunnel: w478 -> [_ w496]
              tunnel: w477 -> [w486 w491]
              tunnel: [w486 w490] -> w476
              tunnel: [w485 w489] -> w475
              tunnel: w474 -> [w485 _]
              frame Default {
                n192 = One Button Dialog(message="That tag is already\npresent in the list.") -> ()  [unwired: 1 in, 1 out]
              }
              frame -1 {
                n193 = Build Array (concatenate)(w493, w500) -> (w498:string[])
                n194 = Array Size(array=w493) -> (size(s)=w494:i32)
                n195 = Bundle By Name(cluster=w499, "tags"=w498) -> (w495:T8)
                n196 = local write "tags"(w494) -> ()
                n197 = Build Array (concatenate)(t_DataLog_Tag_Subset_Editor_States."update lists" ("states"), w491) -> (w490:T3[])
                n198 = Replace Array Subset(array=w489, new element=w495, index=w496) -> (w497:T8[])
              }
            }
          }
        }
      }
      frame "add tags" {
        n199 = call "ui_DataLog Query Tags.vi"("prompt"="Select  tags to add", "database"=w503) -> ("OK?"=w511:bool, "tag"=w510:string[])  [unwired: 12 in]
        n200 = case "OKed?" shown="True" w511 {
          tunnel: w513 -> [w516 w522]
          tunnel: [w516 w530] -> w512
          tunnel: w510 -> [_ w532]
          tunnel: w505 -> [w515 w528]
          tunnel: [w515 w527] -> w504
          tunnel: [w514 w520] -> w502
          tunnel: w501 -> [w514 w517]
          frame False {
          }
          frame True {
            n201 = local read "subsets"() -> (w529:i32)
            n202 = Index Array(array=w522, index=w529) -> (element=w531:T8)
            n203 = Unbundle By Name(w531) -> ("tags"=w533:string[])
            n204 = for "remove tags already present" {
              tunnel: w533 -> [w545]
              tunnel: w532 -> [w541] mode=indexing
              shift-right: [w540] -> w521
              shift-left: string[] [] -> [w542]
              n205 = Search 1D Array(1D array=w545, element=w541) -> (index of element=w544:i32)  [unwired: 1 in]
              n206 = Less Than 0?(x=w544) -> (x < 0?=w543:bool)
              n207 = case shown="True" w543 {
                tunnel: w542 -> [w546 w549]
                tunnel: w541 -> [_ w548]
                tunnel: [w546 w547] -> w540
                frame False {
                }
                frame True {
                  n208 = Build Array (concatenate)(w549, w548) -> (w547:string[])
                }
              }
            }
            n209 = Build Array (concatenate)(w533, w521) -> (w526:string[])
            n210 = Array Size(array=w521) -> (size(s)=w519:i32)
            n211 = Bundle By Name(cluster=w531, "tags"=w526) -> (w525:T8)
            n212 = Build Array (concatenate)(t_DataLog_Tag_Subset_Editor_States."update lists" ("states"), w528) -> (w527:T3[])
            n213 = Not Equal To 0?(x=w519) -> (x != 0?=w518:bool)
            n214 = case shown="True" w518 {
              tunnel: [w535 w539] -> w530
              tunnel: w529 -> [_ w538]
              tunnel: w525 -> [_ w537]
              tunnel: w522 -> [w535 w536]
              tunnel: [w534 w536] -> w520
              tunnel: w517 -> [w534 _]
              frame False {
              }
              frame True {
                n215 = Replace Array Subset(array=w536, new element=w537, index=w538) -> (w539:T8[])
              }
            }
          }
        }
      }
      frame "remove tag" {
        n216 = local read "subsets"() -> (w553:i32)
        n217 = Index Array(array=w558, index=w553) -> (element=w563:T8)
        n218 = Unbundle By Name(w563) -> ("tags"=w562:string[])
        n219 = local read "tags"() -> (w550:i32)
        n220 = Delete From Array(array=w562, index=w550) -> (array with subset deleted=w551:string[])  [unwired: 1 in, 1 out]
        n221 = Bundle By Name(cluster=w563, "tags"=w551) -> (w561:T8)
        n222 = Array Size(array=w551) -> (size(s)=w555:i32)
        n223 = Decrement(x=w555) -> (x-1=w554:i32)
        n224 = Replace Array Subset(array=w558, new element=w561, index=w553) -> (w556:T8[])
        n225 = Max & Min(x=w550, y=w554) -> (min(x,y)=w552:i32)  [unwired: 1 out]
        n226 = Not Equal?(x=w556, y=w558) -> (x != y?=w557:bool)
        n227 = local write "tags"(w552) -> ()
        n228 = Select(t=w558, s=w557, f=w559) -> (s? t:f=w560:T8[])
        n229 = Build Array (concatenate)(t_DataLog_Tag_Subset_Editor_States."update lists" ("states"), w570) -> (w569:T3[])
      }
      frame "sort tags" {
        # "avoid LV7 bug"
        n230 = local read "subsets"() -> (w591:i32)
        n231 = Index Array(array=w572, index=w591) -> (element=w592:T8)
        n232 = local read "tags"() -> (w579:i32)
        n233 = Unbundle By Name(w592) -> ("tags"=w580:string[])
        n234 = for "prepend for sorting" {
          tunnel: w580 -> [w596] mode=indexing
          tunnel: [w598] -> w586 mode=indexing
          # "Lower case. This makes\nthe sort case insensitive\nand gives the underscore\na lower priority so that\nmeta tags group with\ntheir base tag."
          n235 = To Lower Case(string=w596) -> (all lower case string=w597:string)
          n236 = Bundle(w597, "String"=w596) -> (w598:cluster{string, "String":string})  [unwired: 1 in]
        }
        n237 = Index Array(array=w580, index=w579) -> (element=w578:string)
        n238 = Sort 1D Array(array=w586) -> (sorted array=w587:cluster{string, "String":string}[])
        n239 = Sort 1D Array(array=w587) -> (sorted array=w585:cluster{string, "String":string}[])
        n240 = for {
          tunnel: w585 -> [w595] mode=indexing
          tunnel: [w594] -> w576 mode=indexing
          n241 = Unbundle(w595) -> ("String"=w594:string)  [unwired: 1 out]
        }
        n242 = Bundle By Name(cluster=w592, "tags"=w576) -> (w590:T8)
        n243 = Search 1D Array(1D array=w576, element=w578) -> (index of element=w577:i32)  [unwired: 1 in]
        n244 = Replace Array Subset(array=w572, new element=w590, index=w591) -> (w573:T8[])
        n245 = local write "tags"(w577) -> ()
        n246 = Not Equal?(x=w573, y=w572) -> (x != y?=w571:bool)
        n247 = Build Array (concatenate)(t_DataLog_Tag_Subset_Editor_States."update lists" ("states"), w593) -> (w589:T3[])
        n248 = Select(t=w572, s=w571, f=w574) -> (s? t:f=w575:T8[])
      }
      frame "update lists" {
        n249 = Not Equal?(x=w603, y=w604) -> (x != y?=w600:bool)
        n250 = Index Array(array=w603, index="subsets") -> (element=w611:T8)
        n251 = for {
          tunnel: [w626] -> w609 mode=indexing
          tunnel: w603 -> [w625] mode=indexing
          n252 = Unbundle By Name(w625) -> ("name"=w626:string)
        }
        n253 = Unbundle By Name(w611) -> ("tags"=w610:string[])
        n254 = property on="tags" class="LstBox (strict)"("Item Names"=w610) -> ()  [unwired: 2 in, 2 out]
        n255 = property on="subsets" class="LstBox (strict)"("Item Names"=w609) -> ()  [unwired: 2 in, 2 out]
        n256 = Not Equal?(x=w602, y=w600) -> (x != y?=w601:bool)
        n257 = case "modified status changed?" shown="True" w601 {
          tunnel: w600 -> [_ w616]
          frame False {
          }
          frame True {
            n258 = property class="VI"() -> ("Front Panel Window:Title"=w615:string)  [unwired: 2 in, 2 out]
            n259 = case "modified?" shown="True" w616 {
              tunnel: w615 -> [w620 w624]
              tunnel: [w621 w622] -> w614
              frame False {
                n260 = String Length(string=w620) -> (length=w619:i32)
                n261 = Subtract(x=w619, y=2) -> (x-y=w618:i32)
                n262 = String Subset(string=w620, length (rest)=w618) -> (substring=w621:string)  [unwired: 1 in]
              }
              frame True {
                n263 = Concatenate Strings(w624, " *" ("string")) -> (w622:string)
              }
            }
            n264 = property class="VI"("Front Panel Window:Title"=w614) -> ()  [unwired: 2 in, 2 out]
          }
        }
        n265 = Build Array (concatenate)(t_DataLog_Tag_Subset_Editor_States."ablement" ("states"), w613) -> (w606:T3[])
      }
      frame "ablement" {
        w631 = u8 2 items=["enabled", "disabled", "grayed"] ("disabled state")
        n266 = property on="tags" class="LstBox (strict)"() -> ("Item Names"=w653:string[])  [unwired: 2 in, 2 out]
        n267 = case shown="\"unlocked\", \"live\"" w654 {
          tunnel: [w658 w659] -> w632
          frame "locked", "mirrored" {
            w658 = u8 2 items=["enabled", "disabled", "grayed"] ("disabled state")
          }
          frame "unlocked", "live" {
            w659 = u8 0 items=["enabled", "disabled", "grayed"] ("disabled state")
          }
        }
        n268 = Array Size(array=w653) -> (size(s)=w639:i32)
        n269 = Greater Or Equal To 0?(x="tags") -> (x >= 0?=w651:bool)
        n270 = Greater Than 0?(x=w639) -> (x > 0?=w642:bool)
        n271 = local read "subsets"() -> (w648:i32)
        n272 = And(x=w642, y=w651) -> (x .and. y?=w650:bool)
        n273 = Array Size(array=w628) -> (size(s)=w637:i32)
        n274 = Greater Than 0?(x=w637) -> (x > 0?=w644:bool)
        n275 = Greater Or Equal To 0?(x=w648) -> (x >= 0?=w647:bool)
        n276 = Greater?(x=w637, y=1) -> (0:w636:bool)
        n277 = Greater?(x=w639, y=1) -> (0:w641:bool)
        n278 = And(x=w644, y=w647) -> (x .and. y?=w629:bool)
        n279 = Select(t=w632, s=w636, f=w631) -> (s? t:f=w635:u8)
        n280 = Select(t=w632, s=w641, f=w631) -> (s? t:f=w643:u8)
        n281 = Not Equal?(x=w628, y=w630) -> (x != y?=w627:bool)
        n282 = property on="new subset" class="Bool"("Disabled"=w632) -> ()  [unwired: 2 in, 2 out]
        n283 = property on="sort subsets" class="Bool"("Disabled"=w635) -> ()  [unwired: 2 in, 2 out]
        n284 = property on="sort tags" class="Bool"("Disabled"=w643) -> ()  [unwired: 2 in, 2 out]
        n285 = Select(t=w632, s=w650, f=w631) -> (s? t:f=w649:u8)
        n286 = Select(t=w632, s=w629, f=w631) -> (s? t:f=w634:u8)
        n287 = Select(t=w632, s=w646, f=w631) -> (s? t:f=w645:u8)
        n288 = Select(t=w632, s=w627, f=w631) -> (s? t:f=w633:u8)
        n289 = property on="remove tag" class="Bool"("Disabled"=w649) -> ()  [unwired: 2 in, 2 out]
        n290 = property on="rename subset" class="Bool"("Disabled"=w634) -> ()  [unwired: 2 in, 2 out]
        n291 = property on="delete subset" class="Bool"("Disabled"=w634) -> ()  [unwired: 2 in, 2 out]
        n292 = property on="add tag" class="Bool"("Disabled"=w634) -> ()  [unwired: 2 in, 2 out]
        n293 = property on="add multiple tags" class="Bool"("Disabled"=w634) -> ()  [unwired: 2 in, 2 out]
        n294 = property on="save subsets" class="Bool"("Disabled"=w645) -> ()  [unwired: 2 in, 2 out]
        n295 = property on="undo" class="Bool"("Disabled"=w633) -> ()  [unwired: 2 in, 2 out]
      }
      frame "resize" {
        n296 = stacked-sequence {
          frame #0 {
            n297 = property class="VI"() -> ("Front Panel"=w667:refnum<vi>)  [unwired: 2 in, 2 out]
            n298 = property class="Pnl"(reference=w667, "Defer Panel Updates"=TRUE) -> ()  [unwired: 1 in, 2 out]
          }
          frame #1 {
            n299 = property on="subsets" class="LstBox (strict)"() -> ("Position:Top"=w692:i32, "Position:Left"=w689:i32, "Bounds:Width"=w688:u32)  [unwired: 2 in, 2 out]
            n300 = property on="sort subsets" class="Bool"() -> ("Position:Left"=w678:i32, "Bounds:Width"=w677:u32)  [unwired: 2 in, 2 out]
            n301 = property on="tags" class="LstBox (strict)"() -> ("Position:Top"=w682:i32, "Position:Left"=w684:i32, "Bounds:Width"=w685:u32)  [unwired: 2 in, 2 out]
            n302 = property on="sort tags" class="Bool"() -> ("Position:Left"=w679:i32, "Bounds:Width"=w680:u32)  [unwired: 2 in, 2 out]
            n303 = To Long Integer(number=w688) -> (32bit integer=w687:i32)
            n304 = To Long Integer(number=w677) -> (32bit integer=w676:i32)
            n305 = To Long Integer(number=w685) -> (32bit integer=w686:i32)
            n306 = To Long Integer(number=w680) -> (32bit integer=w681:i32)
            n307 = Add(x=w689, y=w687) -> (x+y=w675:i32)
            n308 = Add(x=w678, y=w676) -> (x+y=w674:i32)
            n309 = Add(x=w684, y=w686) -> (x+y=w670:i32)
            n310 = Add(x=w679, y=w681) -> (x+y=w669:i32)
            n311 = Subtract(x=w692, y=7) -> (x-y=w690:i32)
            n312 = Subtract(x=w682, y=7) -> (x-y=w672:i32)
            n313 = Subtract(x=w675, y=w674) -> (x-y=w673:i32)
            n314 = Subtract(x=w670, y=w669) -> (x-y=w671:i32)
            n315 = stacked-sequence {
              tunnel: w690 -> [w712 w716 w720 w724]
              tunnel: w673 -> [w709 w713 w717 w721]
              frame #0 {
                n316 = property on="new subset" class="Bool"() -> ("Position:Left"=w711:i32)  [unwired: 2 in, 2 out]
                n317 = Add(x=w711, y=w709) -> (x+y=w710:i32)
                n318 = property on="new subset" class="Bool"("Position:Top"=w712, "Position:Left"=w710) -> ()  [unwired: 2 in, 2 out]
              }
              frame #1 {
                n319 = property on="rename subset" class="Bool"() -> ("Position:Left"=w715:i32)  [unwired: 2 in, 2 out]
                n320 = Add(x=w715, y=w713) -> (x+y=w714:i32)
                n321 = property on="rename subset" class="Bool"("Position:Top"=w716, "Position:Left"=w714) -> ()  [unwired: 2 in, 2 out]
              }
              frame #2 {
                n322 = property on="delete subset" class="Bool"() -> ("Position:Left"=w719:i32)  [unwired: 2 in, 2 out]
                n323 = Add(x=w719, y=w717) -> (x+y=w718:i32)
                n324 = property on="delete subset" class="Bool"("Position:Top"=w720, "Position:Left"=w718) -> ()  [unwired: 2 in, 2 out]
              }
              frame #3 {
                n325 = property on="sort subsets" class="Bool"() -> ("Position:Left"=w723:i32)  [unwired: 2 in, 2 out]
                n326 = Add(x=w723, y=w721) -> (x+y=w722:i32)
                n327 = property on="sort subsets" class="Bool"("Position:Top"=w724, "Position:Left"=w722) -> ()  [unwired: 2 in, 2 out]
              }
            }
            n328 = stacked-sequence {
              tunnel: w672 -> [w696 w700 w704 w708]
              tunnel: w671 -> [w693 w697 w701 w705]
              frame #0 {
                n329 = property on="add tag" class="Bool"() -> ("Position:Left"=w695:i32)  [unwired: 2 in, 2 out]
                n330 = Add(x=w695, y=w693) -> (x+y=w694:i32)
                n331 = property on="add tag" class="Bool"("Position:Top"=w696, "Position:Left"=w694) -> ()  [unwired: 2 in, 2 out]
              }
              frame #1 {
                n332 = property on="add multiple tags" class="Bool"() -> ("Position:Left"=w699:i32)  [unwired: 2 in, 2 out]
                n333 = Add(x=w699, y=w697) -> (x+y=w698:i32)
                n334 = property on="add multiple tags" class="Bool"("Position:Top"=w700, "Position:Left"=w698) -> ()  [unwired: 2 in, 2 out]
              }
              frame #2 {
                n335 = property on="remove tag" class="Bool"() -> ("Position:Left"=w703:i32)  [unwired: 2 in, 2 out]
                n336 = Add(x=w703, y=w701) -> (x+y=w702:i32)
                n337 = property on="remove tag" class="Bool"("Position:Top"=w704, "Position:Left"=w702) -> ()  [unwired: 2 in, 2 out]
              }
              frame #3 {
                n338 = property on="sort tags" class="Bool"() -> ("Position:Left"=w707:i32)  [unwired: 2 in, 2 out]
                n339 = Add(x=w707, y=w705) -> (x+y=w706:i32)
                n340 = property on="sort tags" class="Bool"("Position:Top"=w708, "Position:Left"=w706) -> ()  [unwired: 2 in, 2 out]
              }
            }
          }
          frame #2 {
            n341 = property class="VI"() -> ("Front Panel"=w726:refnum<vi>)  [unwired: 2 in, 2 out]
            n342 = property class="Pnl"(reference=w726, "Defer Panel Updates"=FALSE) -> ()  [unwired: 1 in, 2 out]
          }
        }
      }
      frame "initialize" {
        n343 = while "rebuild init list on first run or after load or recompile" {
          shift-left: _ -> [w736]
          shift-right: [w735] -> w733
          stop <- FALSE continue-if-true
          n344 = Array Size(array=w736) -> (size(s)=w737:i32)
          n345 = case shown="0" w737 {
            tunnel: [w738 w758] -> w735
            tunnel: w736 -> [w739 w758]
            frame 0 {
              n346 = while {
                shift-left: w739 -> [w748]
                shift-right: [w746] -> w738
                shift-left: _ -> [w750]
                shift-right: [w745] -> _
                i -> [w753]
                stop <- w741 continue-if-true
                n347 = To Unsigned Word Integer(number=w753) -> (unsigned 16bit integer=w751:u16)
                n348 = Type Cast(type=t_DataLog_Tag_Subset_Editor_States."initialize" ("states"), x=w751) -> (*(type *) &x=w747:T3)
                n349 = Format Into String(format string="%s" ("Format String"), w747) -> (resulting string=w745:string)  [unwired: 2 in, 1 out]
                n350 = Not Equal?(x=w745, y=w750) -> (x != y?=w741:bool)
                n351 = Match Pattern(string=w745, regular expression="^init ") -> (offset past match=w743:i32)  [unwired: 1 in, 3 out]
                n352 = Greater Or Equal To 0?(x=w743) -> (x >= 0?=w742:bool)
                n353 = And(x=w742, y=w741) -> (x .and. y?=w740:bool)
                n354 = case shown="True" w740 {
                  tunnel: w748 -> [w754 w757]
                  tunnel: w747 -> [_ w756]
                  tunnel: [w754 w755] -> w746
                  frame False {
                  }
                  frame True {
                    n355 = Build Array (concatenate)(w757, w756) -> (w755:T3[])
                  }
                }
              }
            }
            frame Default {
            }
          }
        }
      }
      frame "init refs" {
        w782 = T3[] [enum."cleanup"] items=["empty queue", "set database", "load subsets", "save subsets", "new subset", "rename subset", "delete subset", "sort subsets", "add tag", "add tags", "remove tag", "sort tags", "update lists", "ablement", "resize", "initialize", "init refs", "init databases", "init access", "init persist", "cleanup", "stop"] ("Array Constant")
        n356 = call "obj_ClientSrv Connection State.vi"("machine{connect}/VI{get state} name (local/no path resolution)"="DataLog Databases_srv.vi") -> ("server app ref"=w765:refnum<vi>, "resolved server path"=w766:path, "error out"=w767:errorcluster)  [unwired: 7 in, 5 out]
        n357 = local read "databases"() -> (w769:T1)
        n358 = stacked-sequence {
          tunnel: [w811] -> w768
          tunnel: [w810] -> w770
          tunnel: w767 -> [w809]
          tunnel: w765 -> [w808]
          tunnel: w766 -> [w807]
          tunnel: w769 -> [w806]
          frame #0 {
            # "avoid LV8 complaints"
            n359 = Path to Array of Strings(0:w807) -> (2:w812:string[])  [unwired: 1 out]
            n360 = Array Size(array=w812) -> (size(s)=w813:i32)
            n361 = case shown="1" w813 {
              tunnel: w807 -> [w820 w826]
              tunnel: w808 -> [w818 w825]
              tunnel: [w816 w821] -> w811
              tunnel: [w814 w824] -> w810
              tunnel: w806 -> [w815 w823]
              tunnel: w809 -> [w817 w822]
              frame 1 {
                n362 = Path To String(path=w820) -> (string=w819:string)
                n363 = Open VI Reference(type specifier VI Refnum (for type only)=w815, application reference (local)=w818, vi path=w819, error in (no error)=w817) -> (vi reference=w816:T1, error out=w814:errorcluster)  [unwired: 2 in]
              }
              frame Default {
                n364 = Open VI Reference(type specifier VI Refnum (for type only)=w823, application reference (local)=w825, vi path=w826, error in (no error)=w822) -> (vi reference=w821:T1, error out=w824:errorcluster)  [unwired: 2 in]
              }
            }
          }
        }
        "databases" <- w768
        n365 = call "Library Open VI Ref Error Clarifier.vi"("VI path"=w766, "called VI error (no error)"=w770) -> ("error out"=w775:errorcluster)  [unwired: 13 in]
        n366 = call "obj_ClientSrv Connection State.vi"("machine{connect}/VI{get state} name (local/no path resolution)"="DataLog Database Infos_srv.vi", "error in (no error)"=w775) -> ("server app ref"=w762:refnum<vi>, "resolved server path"=w761:path, "error out"=w763:errorcluster)  [unwired: 6 in, 5 out]
        n367 = local read "database infos"() -> (w760:T2)
        n368 = stacked-sequence {
          tunnel: [w790] -> w759
          tunnel: [w789] -> w764
          tunnel: w763 -> [w788]
          tunnel: w762 -> [w787]
          tunnel: w761 -> [w786]
          tunnel: w760 -> [w785]
          frame #0 {
            # "avoid LV8 complaints"
            n369 = Path to Array of Strings(0:w786) -> (2:w791:string[])  [unwired: 1 out]
            n370 = Array Size(array=w791) -> (size(s)=w792:i32)
            n371 = case shown="1" w792 {
              tunnel: w786 -> [w799 w805]
              tunnel: w787 -> [w797 w804]
              tunnel: [w795 w800] -> w790
              tunnel: [w793 w803] -> w789
              tunnel: w785 -> [w794 w802]
              tunnel: w788 -> [w796 w801]
              frame 1 {
                n372 = Path To String(path=w799) -> (string=w798:string)
                n373 = Open VI Reference(type specifier VI Refnum (for type only)=w794, application reference (local)=w797, vi path=w798, error in (no error)=w796) -> (vi reference=w795:T2, error out=w793:errorcluster)  [unwired: 2 in]
              }
              frame Default {
                n374 = Open VI Reference(type specifier VI Refnum (for type only)=w802, application reference (local)=w804, vi path=w805, error in (no error)=w801) -> (vi reference=w800:T2, error out=w803:errorcluster)  [unwired: 2 in]
              }
            }
          }
        }
        "database infos" <- w759
        n375 = call "Library Open VI Ref Error Clarifier.vi"("VI path"=w761, "called VI error (no error)"=w764) -> ("error out"=w779:errorcluster)  [unwired: 13 in]
        n376 = call "Library Log Error to Window.vi"("error in (no error)"=w779) -> ("dup error"=w778:errorcluster)  [unwired: 13 in, 1 out]
        n377 = Select(t=w782, s=w778, f=w783) -> (s? t:f=w784:T3[])
      }
      frame "init databases" {
        w838 = T3[] [enum."cleanup"] items=["empty queue", "set database", "load subsets", "save subsets", "new subset", "rename subset", "delete subset", "sort subsets", "add tag", "add tags", "remove tag", "sort tags", "update lists", "ablement", "resize", "initialize", "init refs", "init databases", "init access", "init persist", "cleanup", "stop"] ("Array Constant")
        n378 = local read "databases"() -> (w835:T1)
        n379 = call "obj_ClientSrv Client Access State.vi"() -> ("certificate"=w842:string, "error out"=w844:errorcluster)  [unwired: 14 in]
        n380 = call-by-ref "?"(reference=w835, error in=w844, "certificate in"=w842) -> (error out=w845:errorcluster, "database names"=w830:string[], 15:"error out"=w843:errorcluster)  [unwired: 13 in, 1 out]
        n381 = call "Library Remote Call Error Merger.vi"("call by reference node error"=w845, "called VI error (no error)"=w843) -> ("error out"=w841:errorcluster)  [unwired: 13 in]
        n382 = property on="database" class="Ring (strict)"(error in=w841, "Value"=0 ("index"), "Strings []"=w830) -> (error out=w840:errorcluster)  [unwired: 1 in, 1 out]
        n383 = call "Library Log Error to Window.vi"("error in (no error)"=w840) -> ("dup error"=w836:errorcluster)  [unwired: 13 in, 1 out]
        n384 = Select(t=w838, s=w836, f=w827) -> (s? t:f=w837:T3[])
      }
      frame "init access" {
        w856 = T3[] [enum."cleanup"] items=["empty queue", "set database", "load subsets", "save subsets", "new subset", "rename subset", "delete subset", "sort subsets", "add tag", "add tags", "remove tag", "sort tags", "update lists", "ablement", "resize", "initialize", "init refs", "init databases", "init access", "init persist", "cleanup", "stop"] ("Array Constant")
        # "Ask for operator access up-front so as\nto prevent observers from wasting time\non editing subsets they cannot save."
        n385 = call "obj_ClientSrv Client Access State.vi"("access level (observer)"=t_ClientSrv_Access_Levels."operator") -> ("error out"=w847:errorcluster)  [unwired: 13 in, 1 out]
        n386 = call "Library Log Error to Window.vi"("error in (no error)"=w847) -> ("dup error"=w853:errorcluster)  [unwired: 13 in, 1 out]
        n387 = Select(t=w856, s=w853, f=w854) -> (s? t:f=w855:T3[])
      }
      frame "init persist" {
        w858 = T3[] [enum."resize", enum."set database", enum."load subsets"] items=["empty queue", "set database", "load subsets", "save subsets", "new subset", "rename subset", "delete subset", "sort subsets", "add tag", "add tags", "remove tag", "sort tags", "update lists", "ablement", "resize", "initialize", "init refs", "init databases", "init access", "init persist", "cleanup", "stop"] ("Array Constant")
        n388 = call "Libary Persist Position and Controls.vi"("action"=enum16{"save", "load"}."load") -> ()  [unwired: 13 in, 2 out]
        n389 = Build Array (concatenate)(w858, w865) -> (w859:T3[])
      }
      frame "cleanup" {
        w883 = T3[] [enum."stop"] items=["empty queue", "set database", "load subsets", "save subsets", "new subset", "rename subset", "delete subset", "sort subsets", "add tag", "add tags", "remove tag", "sort tags", "update lists", "ablement", "resize", "initialize", "init refs", "init databases", "init access", "init persist", "cleanup", "stop"] ("Array Constant")
        n390 = call "obj_Library Session.vi"("method"=t_Library_Session_Methods."delist") -> ()  [unwired: 11 in, 4 out]
        n391 = local read "database infos"() -> (w877:T2)
        n392 = local read "databases"() -> (w875:T1)
        n393 = property class="VI"("Front Panel Window:Title"="Tag Subset Editor") -> (error out=w869:errorcluster)  [unwired: 2 in, 1 out]
        n394 = property on="subsets" class="LstBox (strict)"("Item Names"=string[] []) -> ()  [unwired: 2 in, 2 out]
        n395 = property on="tags" class="LstBox (strict)"("Item Names"=string[] []) -> ()  [unwired: 2 in, 2 out]
        n396 = property on="database" class="Ring (strict)"("Strings []"=string[] []) -> ()  [unwired: 2 in, 2 out]
        n397 = Close Reference(reference=w877) -> ()  [unwired: 1 in, 1 out]
        n398 = Close Reference(reference=w875) -> ()  [unwired: 1 in, 1 out]
        n399 = call "Libary Persist Position and Controls.vi"("action"=enum16{"save", "load"}."save", "error in (no error)"=w869) -> ()  [unwired: 12 in, 2 out]
      }
      frame "stop" {
        n400 = invoke class="VI" method="FP.Close"() -> ()  [unwired: 3 in, 3 out]
      }
    }
  }
